vi "XBrio write test3 (array).vi"() -> ()   [LabVIEW 2013]
uses:
  C:/Program Files (x86)/National Instruments/LabVIEW 2013/examples/Instrument IO/Serial/support/Serial - Settings.ctl
  <vilib>/Instr/_visa.llb/VISA Configure Serial Port (Instr).vi
panel:
  out "appended array":u8[](array[numeric])
  in  "Number being sent 2":u8
  out "String being written in HEX":string
  out "String being written":string
  in  "Number being sent":u8
  out "Bytes being written":u32
  in  "VISA resource name":refnum<visa-resource-name>="COM1"
  in  "delay before read (ms)":u32=500
  out "bytes read":u32
  in  "Serial Settings":T1={"baud rate"=9600, "data bits"=8, "parity"=enum."None", "stop bits"=10, "flow control"=0} {"flow control" items=["None"=0, "XON/XOFF"=1, "RTS/CTS"=2, "DTR/DSR"=4]; "stop bits" items=["1.0"=10, "1.5"=15, "2.0"=20]; "data bits" min=5 max=8 step=1; "baud rate" items=["75"=75, "110"=110, "134"=134, "150"=150, "300"=300, "600"=600, "1200"=1200, "1800"=1800, "2400"=2400, "4800"=4800, "7200"=7200, "9600"=9600, "14400"=14400, "19200"=19200, "28800"=28800, "38400"=38400, "56000"=56000, "57600"=57600, "115200"=115200, "128000"=128000, "230400"=230400]}
  in  "?":bool
  out "Response":string
  out "String to U16":u16[](array[numeric])
  out "IR2":u16
  out "IR1":u16
  out "Encoder1":u16
  out "Encoder2":u16
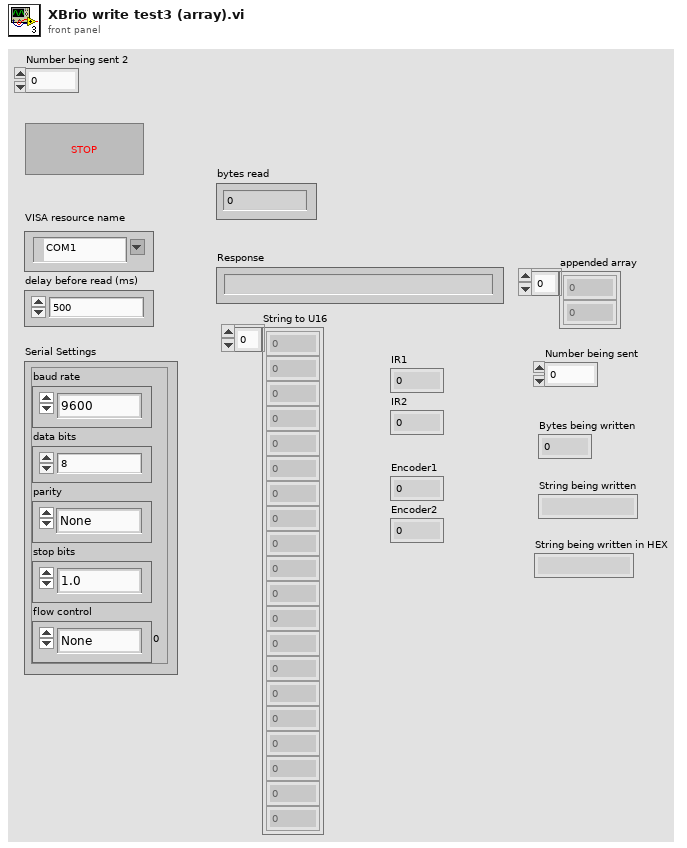
[diagram p1: front panel]
types:
  T1 = typedef "Serial - Settings.ctl" = cluster{"baud rate":u32, "data bits":u16, "parity":enum16{"None", "Odd", "Even", "Mark", "Space"}, "stop bits":u16, "flow control":u16}
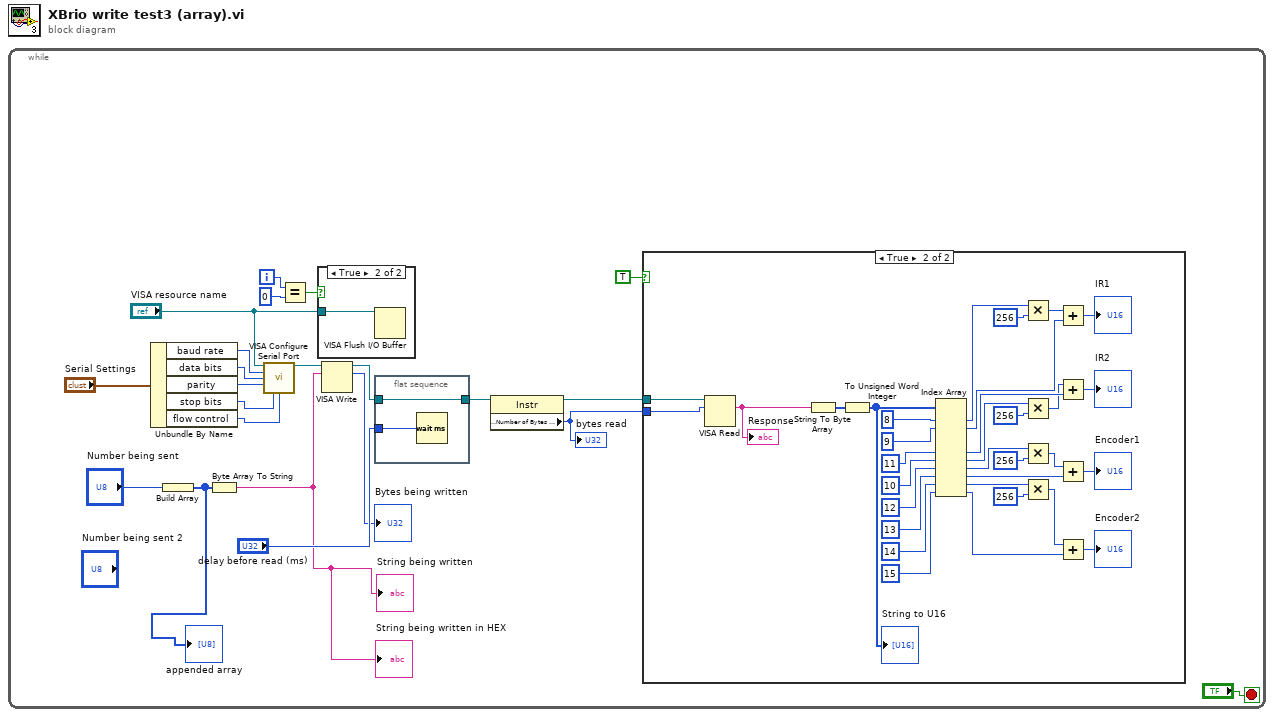
[diagram p0: block diagram]
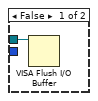
[diagram p2: hidden frame]
diagram:
  n1 = while {
    i -> [w13]
    stop <- "?" stop-if-true
    n2 = Unbundle By Name("Serial Settings") -> ("baud rate"=w20:u32, "data bits"=w19:u16, "parity"=w18:enum16{"None", "Odd", "Even", "Mark", "Space"}, "stop bits"=w17:u16, "flow control"=w16:u16)
    n3 = Build Array("Number being sent") -> (w1:u8[])
    "appended array" <- w1
    n4 = Byte Array To String(unsigned byte array=w1) -> (string=w2:string)
    "String being written" <- w2
    "String being written in HEX" <- w2
    n5 = call-poly "VISA Configure Serial Port"("VISA resource name"="VISA resource name", "baud rate (9600)"=w20, "data bits (8)"=w19, "parity (0:none)"=w18, "stop bits (10: 1 bit)"=w17, "flow control (0:none)"=w16) -> ("VISA resource name out"=w7:refnum<visa-resource-name>)  [unwired: 3 in, 6 out]
    n6 = Equal?(x=w13, y=0) -> (x = y?=w11:bool)
    n7 = case shown="True" w11 {
      tunnel: "VISA resource name" -> [_ w57]
      frame False {
      }
      frame True {
        n8 = VISA Flush I/O Buffer(VISA resource name=w57) -> ()  [unwired: 2 in, 2 out]
      }
    }
    n9 = VISA Write(VISA resource name=w7, write buffer=w2) -> (VISA resource name out=w6:refnum<visa-resource-name>, return count=→"Bytes being written":u32)  [unwired: 1 in, 1 out]
    n10 = flat-sequence {
      tunnel: w6 -> [w58]
      tunnel: [w58] -> w15
      tunnel: "delay before read (ms)" -> [w59]
      frame #0 {
        n11 = Wait (ms)(milliseconds to wait=w59) -> ()  [unwired: 1 out]
      }
    }
    n12 = property class="Instr"(reference=w15) -> (reference out=w8:refnum<visa-resource-name>, "Serial Settings:Number of Bytes at Serial Port"=w9:u32)  [unwired: 1 in, 1 out]
    "bytes read" <- w9
    n13 = case shown="True" TRUE {
      tunnel: w9 -> [_ w25]
      tunnel: w8 -> [w23 w24]
      frame False {
        n14 = VISA Flush I/O Buffer(VISA resource name=w23) -> ()  [unwired: 2 in, 2 out]
      }
      frame True {
        n15 = VISA Read(VISA resource name=w24, byte count=w25) -> (read buffer=w27:string)  [unwired: 1 in, 3 out]
        "Response" <- w27
        n16 = String To Byte Array(string=w27) -> (unsigned byte array=w28:u8[])
        n17 = To Unsigned Word Integer(number=w28) -> (unsigned 16bit integer=w26:u16[])
        "String to U16" <- w26
        n18 = Index Array(array=w26, index #1=8 ("index"), index #2=9 ("index"), index #5=11, index #6=10 ("index"), index #7=12 ("index"), index #8=13 ("index"), index #9=14 ("index"), index #10=15 ("index")) -> (element #1=w36:u16, element #2=w39:u16, element #5=w33:u16, element #6=w31:u16, element #7=w44:u16, element #8=w45:u16, element #9=w51:u16, element #10=w52:u16)  [unwired: 2 in, 2 out]
        n19 = Multiply(x=w36, y=u16 256) -> (x*y=w38:u16)
        n20 = Multiply(x=w31, y=u16 256) -> (x*y=w29:u16)
        n21 = Multiply(x=w44, y=u16 256) -> (x*y=w40:u16)
        n22 = Multiply(x=w51, y=u16 256) -> (x*y=w50:u16)
        n23 = Add(x=w38, y=w39) -> (x+y=→"IR1":u16)
        n24 = Add(x=w29, y=w33) -> (x+y=→"IR2":u16)
        n25 = Add(x=w40, y=w45) -> (x+y=→"Encoder1":u16)
        n26 = Add(x=w50, y=w52) -> (x+y=→"Encoder2":u16)
      }
    }
  }
